vi "ChildModule.Launch.vi"(6 "Dirs":T1, 7 "SW Rev":T2={"AppName"="App Name", "Company"="Company Name", "Version"="0.0.1", "Date"="xx/xx/xx"}, 8 "error in":errorcluster, 10 "Index":i32, 11 "Name":string="ModuleName") -> (0 "error out":errorcluster, 2 "Name Out":string="ModuleName", 3 "VI Ref Out":refnum<vi>)   [LabVIEW 2016]
uses:
  <vilib>/KATE/Module/Public/SW Version Info.ctl
  <vilib>/KATE/Queues/Public/Q.Element.ctl
  <vilib>/KATE/Config/Private/Working Dirs.ctl
  <vilib>/KATE/Module/Public/Module Config.ctl
  <vilib>/KATE/Queues/Queue Utils.lvlib
  <vilib>/KATE/Config/Config Utils.lvlib
  <vilib>/KATE/Module/Module Utils.lvlib
panel:
  in  "Parent Q":refnum<queue>
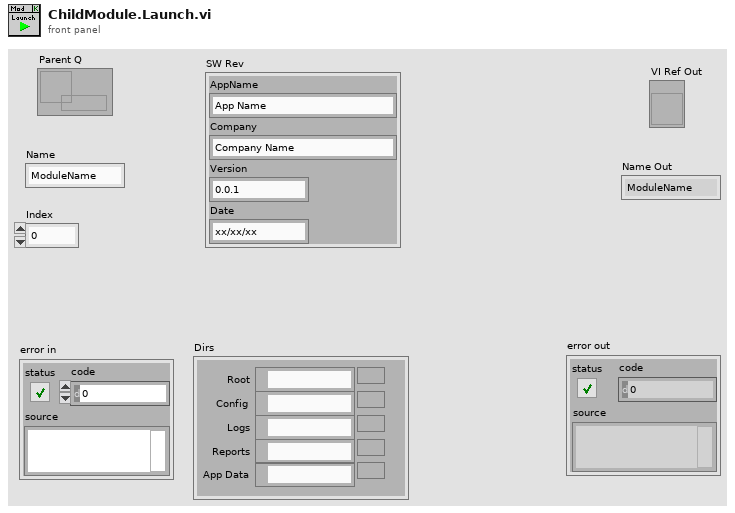
[diagram p1: front panel]
types:
  T1 = typedef "KATE_Lib.lvlib/Config Utils.lvlib/Working Dirs.ctl" = cluster{"Root":path, "Config":path, "Logs":path, "Reports":path, "App Data":path}
  T2 = typedef "KATE_Lib.lvlib/Module Utils.lvlib/SW Version Info.ctl" = cluster{"AppName":string, "Company":string, "Version":string, "Date":string}
  T3 = typedef "KATE_Lib.lvlib/Module Utils.lvlib/Module Config.ctl" = cluster{"Name":string, "Parent Q":refnum<queue>, "Is Child?":bool, "Index":i32, "Dirs":T1}
  T4 = typedef "KATE_Lib.lvlib/Queue Utils.lvlib/Q.Element.ctl" = cluster{"Cmd":string, "Sub":string, "Data1":variant, "Data2":variant}
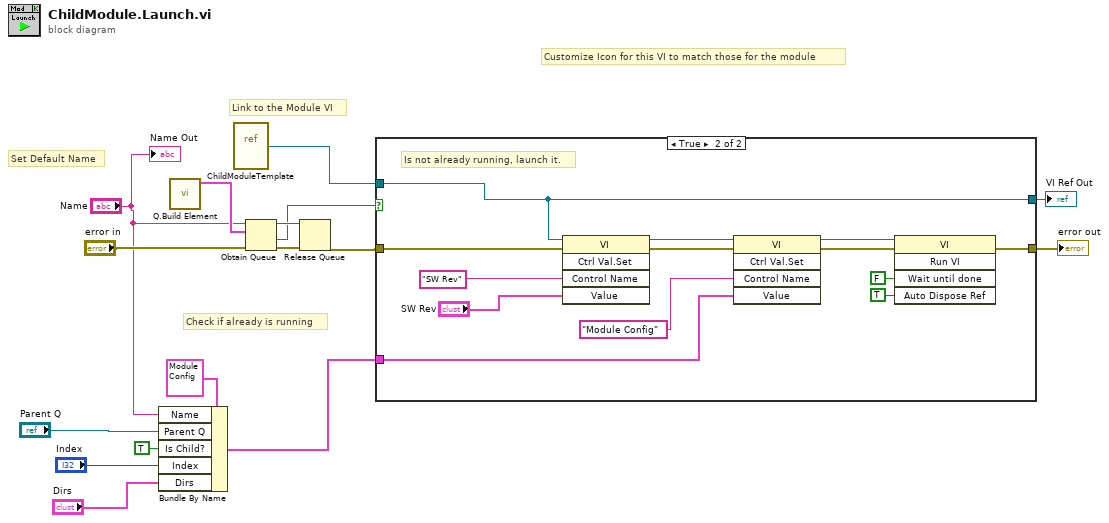
[diagram p0: block diagram]
diagram:
  # "Set Default Name"
  # "Link to the Module VI"
  # "Check if already is running"
  # "Customize Icon for this VI to match those for the module"
  n1 = Bundle By Name(cluster=T3 {"Name"="ModName", "Parent Q"=refnum, "Is Child?"=TRUE, "Index"=0, "Dirs"={"Root"=path "", "Config"=path "C:/ATE/Config", "Logs"=path "C:/ATE/Logs", "Reports"=path "C:/ATE/Reports", "App Data"=path "C:/ProgramData/MAIN"}} ("Module Config"), "Name"="Name", "Parent Q"="Parent Q", "Is Child?"=TRUE, "Index"="Index", "Dirs"="Dirs") -> (w3:T3)
  n2 = call <vilib>:"Q.Build Element.vi"() -> ("Q.Element"=w14:T4)  [unwired: 11 in]
  n3 = vi-ref "ChildModuleTemplate.vi"() -> (w11:refnum<vi>)
  n4 = Obtain Queue(name (unnamed)="Name", element data type=w14, error in (no error)="error in") -> (queue out=w15:refnum<queue>, created new?=w10:bool, error out=w16:errorcluster)  [unwired: 2 in]
  n5 = Release Queue(queue=w15, error in (no error)=w16) -> (error out=w12:errorcluster)  [unwired: 1 in, 2 out]
  n6 = case shown="True" w10 {
    tunnel: [w18 w28] -> w9
    tunnel: w12 -> [w18 w27]
    tunnel: [w17 w26] -> w1
    tunnel: w11 -> [w17 w26]
    tunnel: w3 -> [_ w19]
    frame False {
      # "Is already running.  Do nothing."
    }
    frame True {
      # "Is not already running, launch it."
      n7 = invoke class="VI" method="Ctrl Val.Set"(reference=w26, error in=w27, "Control Name"="SW Rev", "Value"="SW Rev") -> (reference out=w21:refnum<vi>, error out=w22:errorcluster)  [unwired: 1 in, 3 out]
      n8 = invoke class="VI" method="Ctrl Val.Set"(reference=w21, error in=w22, "Control Name"="Module Config", "Value"=w19) -> (reference out=w24:refnum<vi>, error out=w23:errorcluster)  [unwired: 1 in, 3 out]
      n9 = invoke class="VI" method="Run VI"(reference=w24, error in=w23, "Wait until done"=FALSE ("Wait Until Done"), "Auto Dispose Ref"=TRUE ("Auto Dispose Reference")) -> (error out=w28:errorcluster)  [unwired: 1 in, 4 out]
    }
  }
  "error out" <- w9
  "VI Ref Out" <- w1
  "Name Out" <- "Name"
